vi "Get Invalid DMA Configuration.vi"(6 "new bitfile dma channels":T1[](array[typedef]) {"Data Type" format="%.0x"}, 8 "error in (no error)":errorcluster, 10 "old bitfile dma channels":T1[](array[typedef]) {"Data Type" format="%.0x"}, 11 "item ref in":T3 format="%.0x") -> (0 "error out":errorcluster, 2 "invalid dma data channels":T1[](array[typedef]) {"Data Type" format="%.0x"}, 3 "item ref out":T3=18446744073709551615 format="%.0x")   [LabVIEW 2019, in "FPGA Addon System Explorer.lvlib"]
uses:
  FPGA Addon System Explorer.lvlib
  <vilib>/NI VeriStand/Custom Device API/Custom Device Item Ref.ctl
  Addon Shared/Types/DMA Information.ctl
  Addon Shared/Types/FPGA Addon Data Type.ctl
  Addon Shared/FPGA Addon Shared.lvlib
  <vilib>/NI VeriStand/Custom Device API/Custom Device API.lvlib
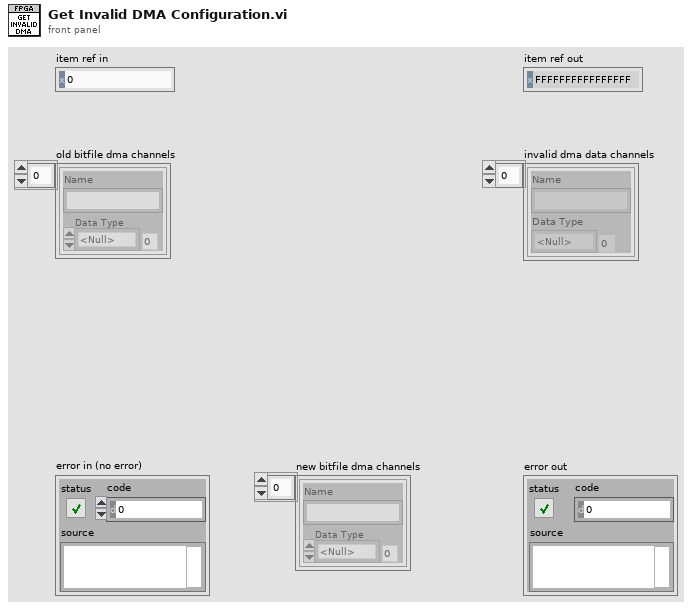
[diagram p1: front panel]
types:
  T1 = typedef "FPGA Addon Shared.lvlib/DMA Information.ctl" = cluster{"Name":string, "Data Type":T2}
  T2 = typedef "FPGA Addon Shared.lvlib/FPGA Addon Data Type.ctl" = enum8{"<Null>", "I8", "I16", "I32", "I64", "U8", "U16", "U32", "U64", "SGL", "Boolean", "Analog PWM In Settings", "Analog PWM In", "Digital PWM In Settings", "Digital PWM In", "Digital PWM Out", "Sine Out", "FXP", "FXP+/-24.5", "FXP+/-16.5", "FXP+/-32.8", "FXP+/-64.32", "FXP+/-16.7", "FXP+/-20.5", "FXP+/-27.5", "FXP+/-32.16", "FXP+16.3", "FXP+18.3", "Digital Static In", "Digital Static Out", "Digital Static In Settings", "Digital WSS Out", "Quad Encoder Settings", "Quad Encoder In", "Group"}
  T3 = typedef "Custom Device API.lvlib/Custom Device Item Ref.ctl" = u64
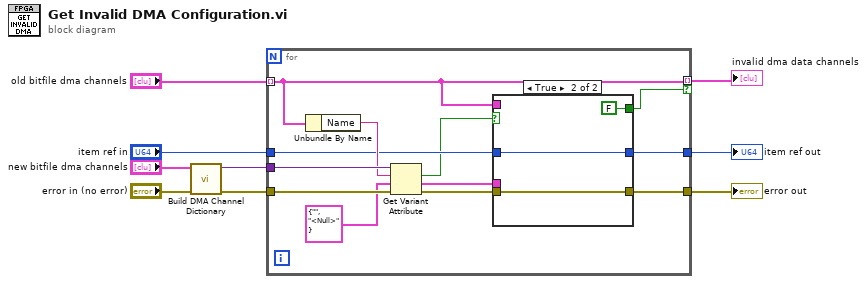
[diagram p0: block diagram]
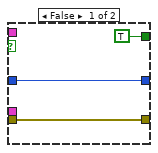
[diagram p2: hidden frame]
diagram:
  n1 = call "Build DMA Channel Dictionary.vi"("error in (no error)"="error in (no error)", "old bitfile dma channels"="new bitfile dma channels") -> ("error out"=w5:errorcluster, "scalar channels dictionary"=w4:variant)  [unwired: 8 in]
  n2 = for {
    tunnel: [w19] -> w8
    tunnel: w5 -> [w21]
    tunnel: w4 -> [w20]
    tunnel: "old bitfile dma channels" -> [w12] mode=indexing
    tunnel: [w12] -> w1 mode=indexing if=w18
    tunnel: "item ref in" -> [w13]
    tunnel: [w17] -> w7
    n3 = Unbundle By Name(w12) -> ("Name"=w16:string)
    n4 = Get Variant Attribute(Variant=w20, name=w16, default value (empty Variant)=T1 {"Name"="", "Data Type"=enum."<Null>"} ("Cluster"), error in=w21) -> (found=w11:bool, value=w14:T1, error out=w15:errorcluster)  [unwired: 1 out]
    n5 = case shown="True" w11 {
      tunnel: w15 -> [w24 w25]
      tunnel: w14 -> [_ _]
      tunnel: w12 -> [_ _]
      tunnel: [w24 w25] -> w19
      tunnel: [TRUE FALSE] -> w18
      tunnel: w13 -> [w23 w26]
      tunnel: [w23 w26] -> w17
      frame False {
      }
      frame True {
      }
    }
  }
  "error out" <- w8
  "item ref out" <- w7
  "invalid dma data channels" <- w1
